vi "ControlLED3.vi"(5 "On?":bool, 7 "All flash?":bool, 8 "Brightness":i16, 9 "Target":i16, 10 "DO Task":refnum<k21>="BlueSimple_DO_All") -> ()   [LabVIEW 2010]
uses:
  Controls/Bits to Write.ctl
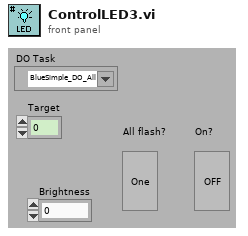
[diagram p1: front panel]
types:
  T1 = typedef "Bits to Write.ctl" = enum16{"LED 1 on", "LED 1 off", "LED 2 on", "LED 2 off", "LED 3 on", "LED 3 off", "LED 4 on", "LED 4 off", "All LEDs on", "All LEDs off", "In trial on", "In trial off", "Buzzer on", "Buzzer off", "Reward on", "Reward off", "Target number", "Trial type preQ on", "Trial type preQ off", "Error on", "Error off", "Trial number", "DBS on", "DBS off", "Sine on", "Sine off", "All Bits On", "All Bits Off", "Init", "Specify mask/pattern"}
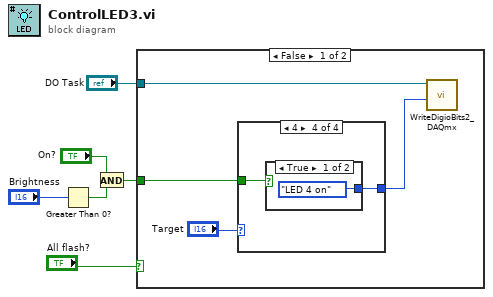
[diagram p0: block diagram]
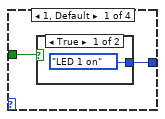
[diagram p2: hidden frame]
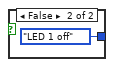
[diagram p3: hidden frame]
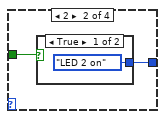
[diagram p4: hidden frame]
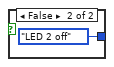
[diagram p5: hidden frame]
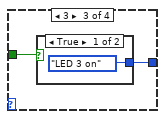
[diagram p6: hidden frame]
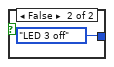
[diagram p7: hidden frame]
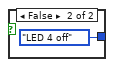
[diagram p8: hidden frame]
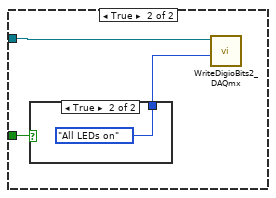
[diagram p9: hidden frame]
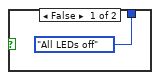
[diagram p10: hidden frame]
diagram:
  n1 = Greater Than 0?(x="Brightness") -> (x > 0?=w4:bool)
  n2 = And(x="On?", y=w4) -> (x .and. y?=w3:bool)
  n3 = case shown="False" "All flash?" {
    tunnel: "DO Task" -> [w8 w28]
    tunnel: w3 -> [w10 w29]
    frame False {
      n4 = case shown="4" "Target" {
        tunnel: w10 -> [w12 w16 w20 w24]
        tunnel: [w11 w15 w19 w23] -> w7
        frame 1, Default {
          n5 = case shown="True" w12 {
            tunnel: [Bits_to_Write."LED 1 on" ("Bits to write") Bits_to_Write."LED 1 off" ("Bits to write")] -> w11
            frame True {
            }
            frame False {
            }
          }
        }
        frame 2 {
          n6 = case shown="True" w16 {
            tunnel: [Bits_to_Write."LED 2 on" ("Bits to write") Bits_to_Write."LED 2 off" ("Bits to write")] -> w15
            frame True {
            }
            frame False {
            }
          }
        }
        frame 3 {
          n7 = case shown="True" w20 {
            tunnel: [Bits_to_Write."LED 3 on" ("Bits to write") Bits_to_Write."LED 3 off" ("Bits to write")] -> w19
            frame True {
            }
            frame False {
            }
          }
        }
        frame 4 {
          n8 = case shown="True" w24 {
            tunnel: [Bits_to_Write."LED 4 on" ("Bits to write") Bits_to_Write."LED 4 off" ("Bits to write")] -> w23
            frame True {
            }
            frame False {
            }
          }
        }
      }
      n9 = call "WriteDigioBits2_DAQmx.vi"("Bits to write"=w7, "DO Task"=w8) -> ()  [unwired: 9 in, 1 out]
    }
    frame True {
      n10 = case shown="True" w29 {
        tunnel: [Bits_to_Write."All LEDs off" ("Bits to write") Bits_to_Write."All LEDs on" ("Bits to write")] -> w27
        frame False {
        }
        frame True {
        }
      }
      n11 = call "WriteDigioBits2_DAQmx.vi"("Bits to write"=w27, "DO Task"=w28) -> ()  [unwired: 9 in, 1 out]
    }
  }
